vi "Polynomial Evaluate.vi"(9 "Data":dbl[](array[numeric]), 10 "Coefficients":dbl[](array[numeric])) -> (1 "Results":dbl[](array[numeric]))   [LabVIEW 2020, in "VolatusData.lvlib" / "DataProcessor.lvclass"]
uses:
  DataProcessor.lvclass
  DataProcessor.lvclass/DataProcessor.ctl
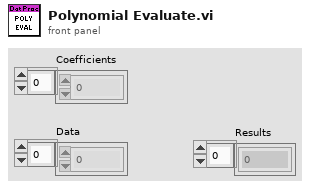
[diagram p1: front panel]
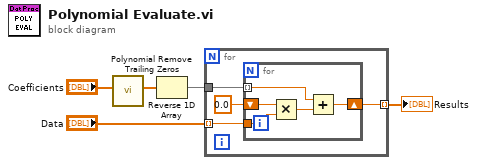
[diagram p0: block diagram]
diagram:
  n1 = call "Polynomial Remove Trailing Zeros.vi"("Coefficients"="Coefficients") -> ("Used Coefficients"=w4:dbl[])  [unwired: 10 in]
  n2 = Reverse 1D Array(array=w4) -> (reversed array=w3:dbl[])
  n3 = for {
    tunnel: w3 -> [w9]
    tunnel: "Data" -> [w8] mode=indexing
    tunnel: [w6] -> w1 mode=indexing
    n4 = for {
      tunnel: w9 -> [w11] mode=indexing
      tunnel: w8 -> [w13]
      shift-right: [w10] -> w6
      shift-left: 0.0 -> [w14]
      n5 = Multiply(x=w14, y=w13) -> (x*y=w12:dbl)
      n6 = Add(x=w11, y=w12) -> (x+y=w10:dbl)
    }
  }
  "Results" <- w1
